vi "checkErrors.vi"(8 "error in (no error)":errorcluster, 11 "TCPCommunicator in":refnum<class "TCPCommunicator.lvclass">) -> (0 "error out":errorcluster, 3 "TCPCommunicator out":refnum<class "TCPCommunicator.lvclass">)   [LabVIEW 2016, in "TCPCommunicator.lvclass"]
uses:
  TCPCommunicator.lvclass
panel:
  out "timeout?":bool
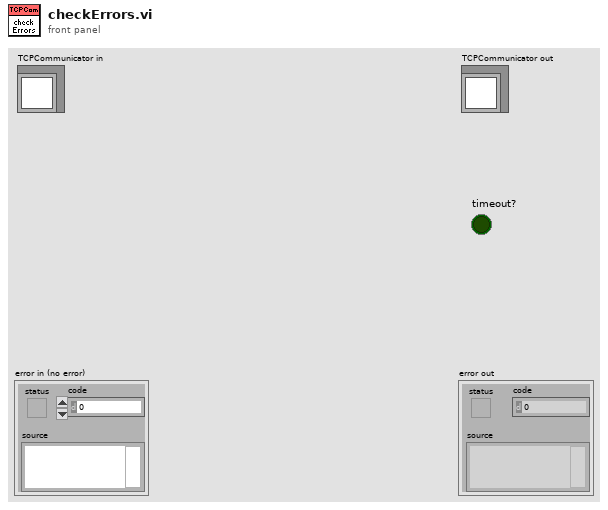
[diagram p1: front panel]
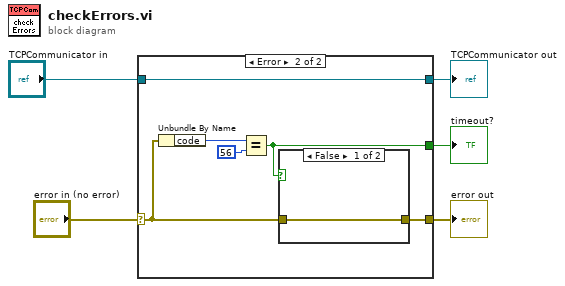
[diagram p0: block diagram]
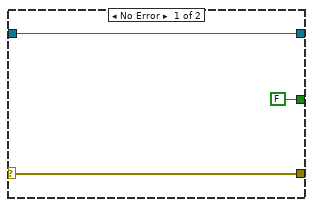
[diagram p2: hidden frame]
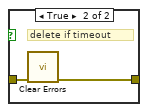
[diagram p3: hidden frame]
diagram:
  n1 = case shown="Error" "error in (no error)" {
    selector: "error in (no error)" -> [w7 w10]
    tunnel: [w7 w9] -> w1
    tunnel: [w8 w14] -> w3
    tunnel: "TCPCommunicator in" -> [w8 w14]
    tunnel: [FALSE ("timeout?") w11] -> w5
    frame No Error {
    }
    frame Error {
      n2 = Unbundle By Name(w10) -> ("code"=w13:i32)
      n3 = Equal?(x=w13, y=56) -> (x = y?=w11:bool)
      n4 = case shown="False" w11 {
        tunnel: w10 -> [w15 w17]
        tunnel: [w15 w16] -> w9
        frame False {
        }
        frame True {
          # "delete if timeout"
          n5 = call <vilib>:"Clear Errors.vi"("error in (no error)"=w17) -> ("error out"=w16:errorcluster)  [unwired: 5 in, 1 out]
        }
      }
    }
  }
  "error out" <- w1
  "TCPCommunicator out" <- w3
  "timeout?" <- w5
